vi "SFC_Shipment.vi"(0 "Traceability 引用句柄":refnum<k24>, 1 "UserNo":string, 2 "ShipType":string, 5 "CartonID":string, 7 "SalesOrder":string, 9 "Model":string, 11 "error in (no error)":errorcluster caption="错误输入（无错误）", 12 "CurCartonShipQTY":i32) -> (4 "Traceability 引用句柄输出":refnum<k24>, 6 "SFC_Shipment":string, 15 "error out":errorcluster caption="错误输出")   [LabVIEW 2014, in "Traceability.lvlib"]
uses:
  D:/webservice/Traceability.dll
  Traceability.dll
  Traceability.lvlib
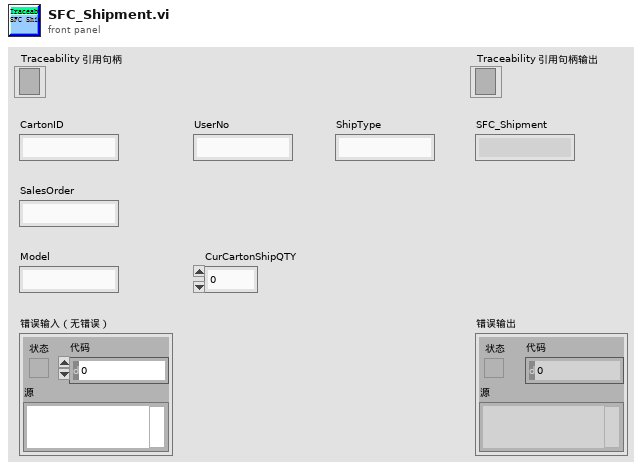
[diagram p1: front panel]
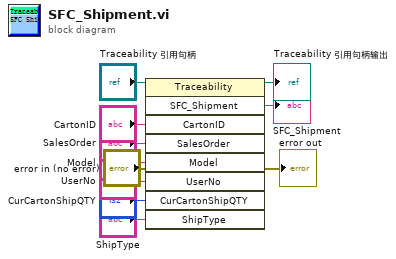
[diagram p0: block diagram]
diagram:
  n1 = invoke class="Traceability" method="SFC_Shipment"(reference="Traceability 引用句柄", error in="error in (no error)", "CartonID"="CartonID", "SalesOrder"="SalesOrder", "Model"="Model", "UserNo"="UserNo", "CurCartonShipQTY"="CurCartonShipQTY", "ShipType"="ShipType") -> (reference out=→"Traceability 引用句柄输出":refnum<k24>, error out=→"error out":errorcluster, "SFC_Shipment"=→"SFC_Shipment":string)  [unwired: 1 in, 6 out]
